vi "counting_tag_scan_direction.vi"(1 "resonant trigger":bool, 5 "initial phase?":bool, 6 "iteration counter initial phase (resonance cycle)":u16, 7 "main phase?":bool, 8 "iterations until end of fly-back scan segment":u16, 9 "iteration counter (resonance cycle)":u16, 10 "x offset fly-forward (iterations)":u16) -> (0 "initial phase? OUT":bool, 2 "iteration counter initial phase (resonance cycle) out":u16, 3 "main phase? OUT":bool, 4 "iteration counter (resonance cycle) out":u16)   [LabVIEW 2010]
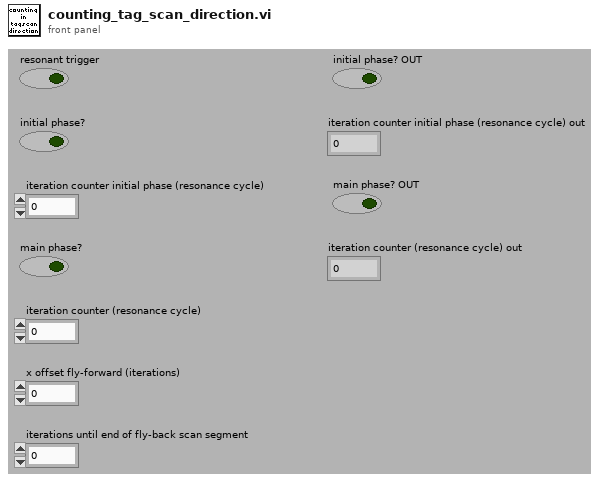
[diagram p1: front panel]
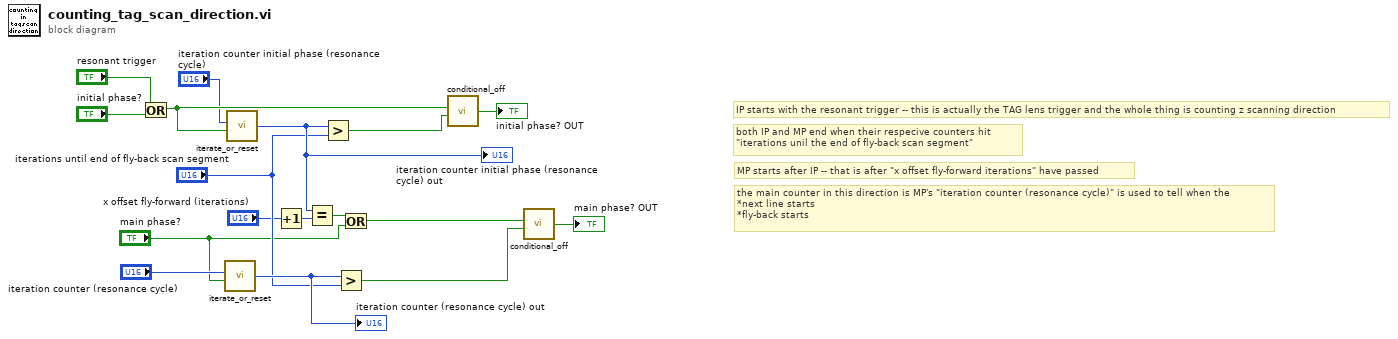
[diagram p0: block diagram]
diagram:
  # "IP starts with the resonant trigger -- this is actually the TAG lens trigger and the whole thing is counting z scanning direction"
  # "the main counter in this direction is MP's \"iteration counter (resonance cycle)\" is used to tell when the\n*next line starts\n*fly-back starts"
  # "MP starts after IP -- that is after \"x offset fly-forward iterations\" have passed"
  # "both IP and MP end when their respecive counters hit \n\"iterations unil the end of fly-back scan segment\""
  n1 = Or(x="resonant trigger", y="initial phase?") -> (x .or. y?=w13:bool)
  n2 = call "iterate_or_reset.vi"("iterate?"="main phase?", "number in"="iteration counter (resonance cycle)") -> ("number out"=w14:u16)  [unwired: 4 in]
  "iteration counter (resonance cycle) out" <- w14
  n3 = call "iterate_or_reset.vi"("iterate?"=w13, "number in"="iteration counter initial phase (resonance cycle)") -> ("number out"=w16:u16)  [unwired: 4 in]
  "iteration counter initial phase (resonance cycle) out" <- w16
  n4 = Increment(x="x offset fly-forward (iterations)") -> (x+1=w9:u16)
  n5 = Equal?(x=w16, y=w9) -> (x = y?=w6:bool)
  n6 = Greater?(x=w16, y="iterations until end of fly-back scan segment") -> (0:w17:bool)
  n7 = Greater?(x=w14, y="iterations until end of fly-back scan segment") -> (0:w7:bool)
  n8 = Or(x=w6, y="main phase?") -> (x .or. y?=w10:bool)
  n9 = call "conditional_off.vi"("switch off?"=w17, "boolean in"=w13) -> ("boolean out"=→"initial phase? OUT":bool)  [unwired: 4 in]
  n10 = call "conditional_off.vi"("switch off?"=w7, "boolean in"=w10) -> ("boolean out"=→"main phase? OUT":bool)  [unwired: 4 in]
